vi "PWM Waveform PD500 Test_v2.vi"(0 "Analysis Leg":i32, 1 "Board Selector":T1, 5 "Active Leg":i32, 9 "Waveform":waveform(dbl)[](array[waveform]), 11 "error in (no error)":errorcluster) -> (4 "Inactive Values":dbl[](array[numeric]), 6 "Active Values":dbl[](array[numeric]), 8 "Error Suppressed?":bool, 15 "error out":errorcluster)   [LabVIEW 2022 SP3]
uses:
  Serial Board Com/Board Select.ctl
  <vilib>/measure/mascope.llb/Pulse Measurements 1 chan.vi
  <vilib>/measure/madcrms.llb/Basic Averaged DC-RMS for 1 Chan.vi
  <vilib>/measure/NI_MAPro.lvlib
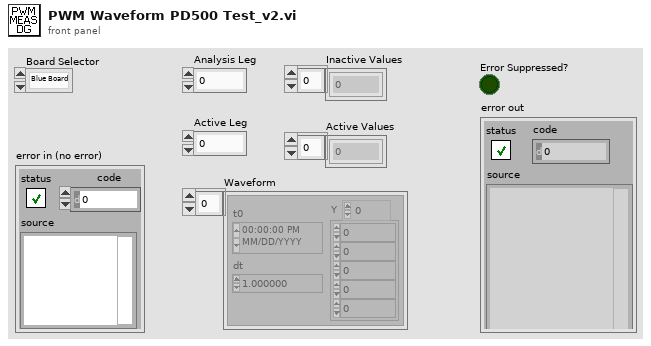
[diagram p1: front panel]
types:
  T1 = typedef "Board Select.ctl" = enum16{"Blue Board", "Green Board"}
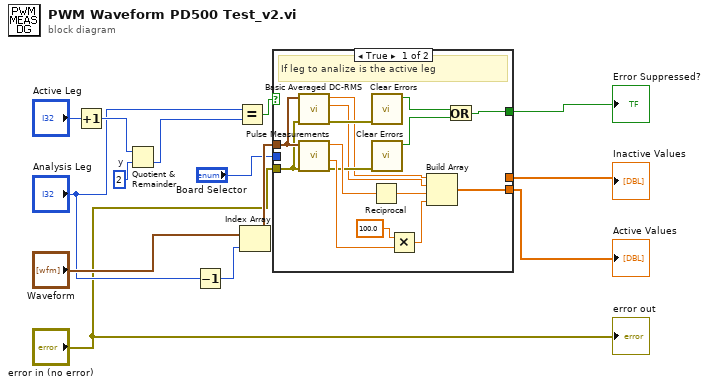
[diagram p0: block diagram]
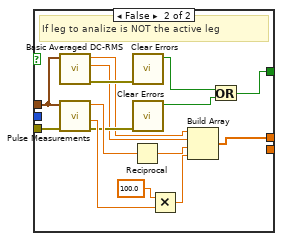
[diagram p2: hidden frame]
diagram:
  w9 = 2  # y
  n1 = Increment(x="Active Leg") -> (x+1=w8:i32)
  n2 = Quotient & Remainder(x=w8, y=w9) -> (floor(x/y)=w6:i32)  [unwired: 1 out]
  n3 = Decrement(x="Analysis Leg") -> (x-1=w4:i32)
  n4 = Equal?(x="Analysis Leg", y=w6) -> (x = y?=w12:bool)
  n5 = Index Array(array="Waveform", index=w4) -> (element=w13:waveform(dbl))
  n6 = case shown="True" w12 {
    tunnel: w13 -> [w24 w39]
    tunnel: "Board Selector" -> [_ _]
    tunnel: [_ w34] -> w10
    tunnel: [w19 _] -> w3
    tunnel: "error in (no error)" -> [w18 w33]
    tunnel: [w15 w30] -> w1
    frame True {
      # "If leg to analize is the active leg"
      n7 = call-poly <vilib>:"Basic Averaged DC-RMS.vi"("error in (no error)"=w18, "signal in"=w24) -> ("error out"=w25:errorcluster, "RMS value"=w22:dbl, "DC value"=w23:dbl)  [unwired: 6 in, 1 out]
      n8 = call-poly <vilib>:"Pulse Measurements.vi"("error in (no error)"=w18, "signal in"=w24) -> ("error out"=w26:errorcluster, "duty cycle"=w28:dbl, "period"=w27:dbl)  [unwired: 5 in, 2 out]
      n9 = Reciprocal(x=w27) -> (1/x=w21:dbl)
      n10 = call <vilib>:"Clear Errors.vi"("error in (no error)"=w25) -> ("specific error cleared?"=w17:bool)  [unwired: 5 in, 1 out]
      n11 = call <vilib>:"Clear Errors.vi"("error in (no error)"=w26) -> ("specific error cleared?"=w16:bool)  [unwired: 5 in, 1 out]
      n12 = Multiply(x=100.0, y=w28) -> (x*y=w20:dbl)
      n13 = Build Array(w23, w22, w21, w20) -> (w19:dbl[])
      n14 = Or(x=w17, y=w16) -> (x .or. y?=w15:bool)
    }
    frame False {
      # "If leg to analize is NOT the active leg"
      n15 = call-poly <vilib>:"Basic Averaged DC-RMS.vi"("signal in"=w39) -> ("error out"=w40:errorcluster, "RMS value"=w37:dbl, "DC value"=w38:dbl)  [unwired: 7 in, 1 out]
      n16 = call-poly <vilib>:"Pulse Measurements.vi"("error in (no error)"=w33, "signal in"=w39) -> ("error out"=w41:errorcluster, "duty cycle"=w43:dbl, "period"=w42:dbl)  [unwired: 5 in, 2 out]
      n17 = Reciprocal(x=w42) -> (1/x=w36:dbl)
      n18 = call <vilib>:"Clear Errors.vi"("error in (no error)"=w40) -> ("specific error cleared?"=w32:bool)  [unwired: 5 in, 1 out]
      n19 = call <vilib>:"Clear Errors.vi"("error in (no error)"=w41) -> ("specific error cleared?"=w31:bool)  [unwired: 5 in, 1 out]
      n20 = Multiply(x=100.0, y=w43) -> (x*y=w35:dbl)
      n21 = Build Array(w38, w37, w36, w35) -> (w34:dbl[])
      n22 = Or(x=w32, y=w31) -> (x .or. y?=w30:bool)
    }
  }
  "Inactive Values" <- w10
  "Active Values" <- w3
  "Error Suppressed?" <- w1
  "error out" <- "error in (no error)"
